vi "display crypted image.vi"(0 "image originale":T1, 1 "X Resolution":i32, 2 "Y Resolution":i32, 7 "red in":i32[](array[numeric]), 9 "green in":i32[](array[numeric]), 11 "blue in":i32[](array[numeric])) -> (8 "image chiffrée":T1)   [LabVIEW 2019]
uses:
  <vilib>/vision/Image Controls.llb/IMAQ Image.ctl
  <vilib>/vision/NI_Vision_Development_Module.lvlib
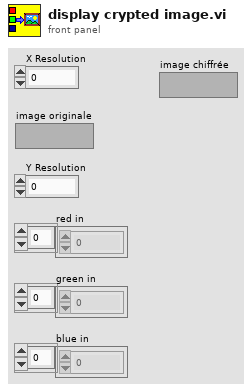
[diagram p1: front panel]
types:
  T1 = typedef "IMAQ Image.ctl" = refnum<image>
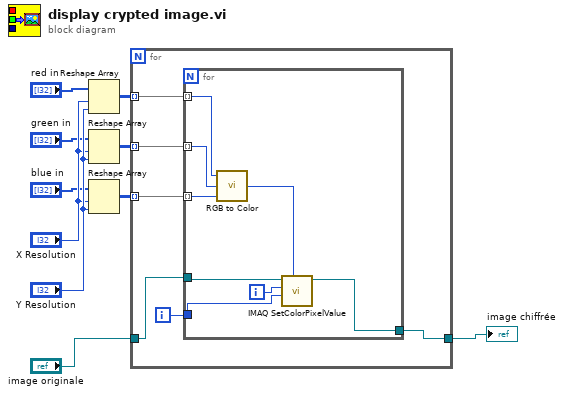
[diagram p0: block diagram]
diagram:
  n1 = Reshape Array("red in", "X Resolution", "Y Resolution") -> (w1:i32[][])
  n2 = Reshape Array("green in", "X Resolution", "Y Resolution") -> (w2:i32[][])
  n3 = Reshape Array("blue in", "X Resolution", "Y Resolution") -> (w3:i32[][])
  n4 = for {
    tunnel: [w15] -> w8
    tunnel: "image originale" -> [w14]
    tunnel: w1 -> [w13] mode=indexing
    tunnel: w2 -> [w12] mode=indexing
    tunnel: w3 -> [w11] mode=indexing
    i -> [w16]
    n5 = for {
      tunnel: w16 -> [w23]
      tunnel: [w21] -> w15
      tunnel: w14 -> [w20]
      tunnel: w13 -> [w19] mode=indexing
      tunnel: w12 -> [w18] mode=indexing
      tunnel: w11 -> [w17] mode=indexing
      i -> [w24]
      n6 = call <vilib>:"RGB to Color.vi"("B"=w17, "G"=w18, "R"=w19) -> ("Color"=w22:u32)
      n7 = call "IMAQ SetColorPixelValue"("Pixel Value (U32)"=w22, "Y Coordinate"=w23, "X Coordinate"=w24, "Image"=w20) -> ("Image Out"=w21:T1)  [unwired: 6 in, 1 out]
    }
  }
  "image chiffrée" <- w8
